vi "Get Length.vi"(8 "error in (no error)":errorcluster caption="错误输入（无错误）", 11 "Scroll Gradient输入":refnum<class "Scroll Gradient.lvclass">) -> (0 "error out":errorcluster caption="错误输出", 2 "Length":i32, 3 "Scroll Gradient输出":refnum<class "Scroll Gradient.lvclass">)   [LabVIEW 2012, in "Picture Box Tools.lvlib" / "Scroll Gradient.lvclass"]
uses:
  Scroll Gradient.lvclass
  Scroll Gradient.lvclass/Scroll Gradient.ctl
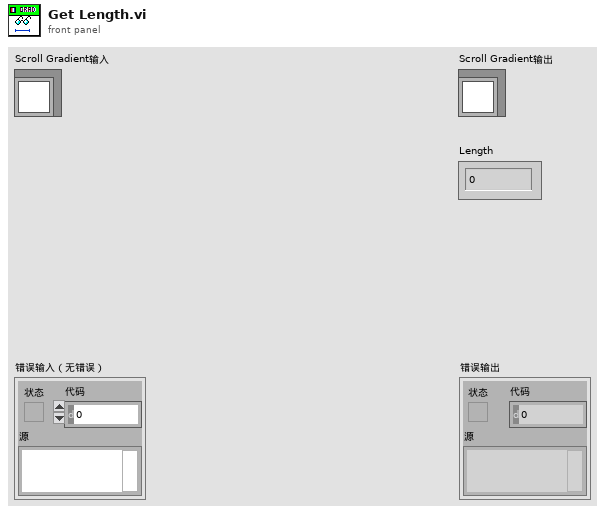
[diagram p1: front panel]
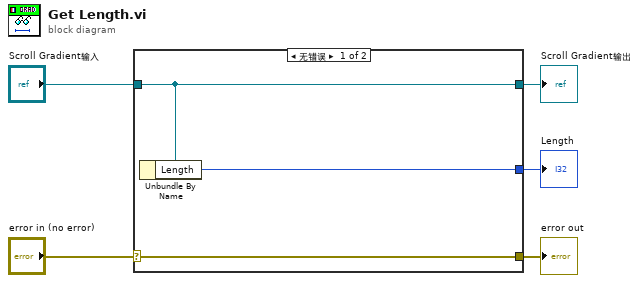
[diagram p0: block diagram]
diagram:
  n1 = case shown="无错误" "error in (no error)" {
    selector: "error in (no error)" -> [w8 w9]
    tunnel: [w8 w9] -> w4
    tunnel: [w7 w10] -> w2
    tunnel: "Scroll Gradient输入" -> [w7 w10]
    tunnel: [w6 _] -> w1
    frame No Error {
      n2 = Unbundle By Name(w7) -> ("Length"=w6:i32)
    }
    frame Error {
    }
  }
  "error out" <- w4
  "Scroll Gradient输出" <- w2
  "Length" <- w1
